vi "Translate - Response JSON Parser.vi"(8 "error in (no error)":errorcluster, 11 "JSON Text":string) -> (0 "error out":errorcluster, 3 "translations":T1(array[cluster]))   [LabVIEW 2015, in "lv-deepl-api.lvlib"]
uses:
  lv-deepl-api.lvlib
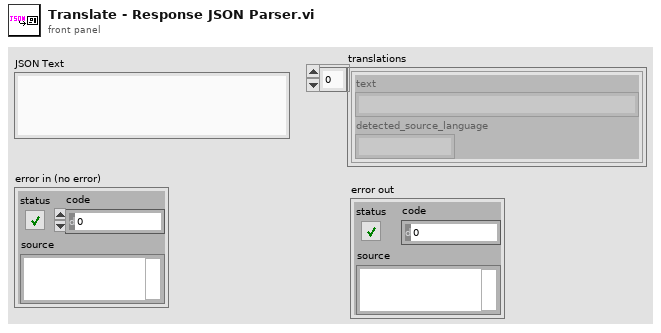
[diagram p1: front panel]
types:
  T1 = cluster{"detected_source_language":string, "text":string}[]
  T2 = cluster{"translations":cluster{"detected_source_language":string, "text":string}[]}
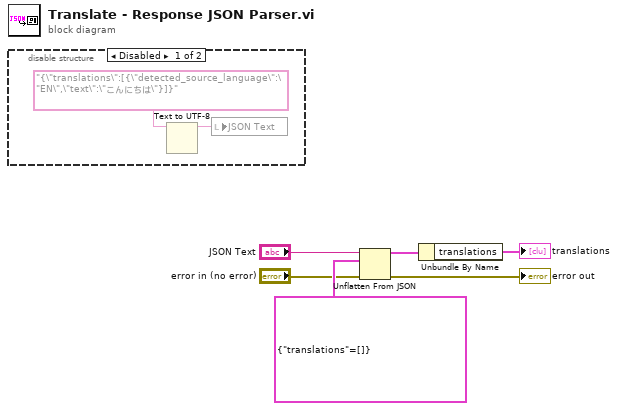
[diagram p0: block diagram]
diagram:
  n1 = disable-structure shown="Disabled" {
    frame Disabled {
      n2 = Text to UTF-8(11:"{\"translations\":[{\"detected_source_language\":\"EN\",\"text\":\"こんにちは\"}]}") -> (3:w7:string)  [unwired: 2 in, 1 out]
      n3 = local write "JSON Text"(w7) -> ()
    }
    frame Enabled {
    }
  }
  n4 = Unflatten From JSON(JSON string="JSON Text", type and defaults=T2 {"translations"=[]}, error in (no error)="error in (no error)") -> (value=w5:T2, error out=→"error out":errorcluster)  [unwired: 4 in]
  n5 = Unbundle By Name(w5) -> ("translations"=→"translations":T1)
